vi "initializeArrayElement.vi"(8 "error in (no error)":errorcluster, 9 "arraySize":u16, 10 "arrayRef":refnum<vi>, 11 "Primitive in":refnum<class "Primitive.lvclass">) -> (0 "error out":errorcluster, 3 "Primitive out":refnum<class "Primitive.lvclass">)   [LabVIEW 2012, in "Primitive.lvclass"]
uses:
  Primitive.lvclass
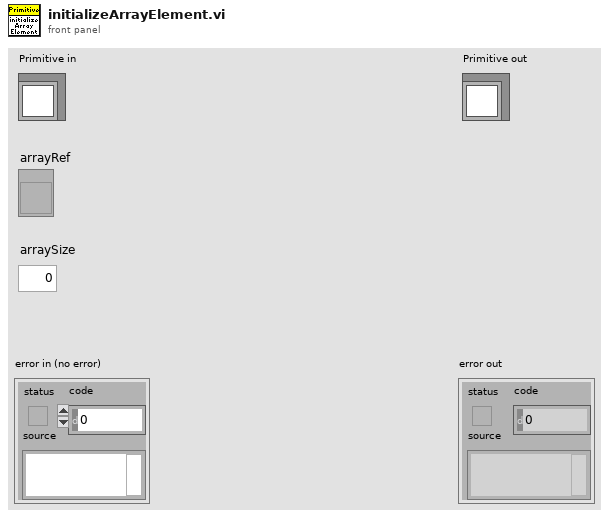
[diagram p1: front panel]
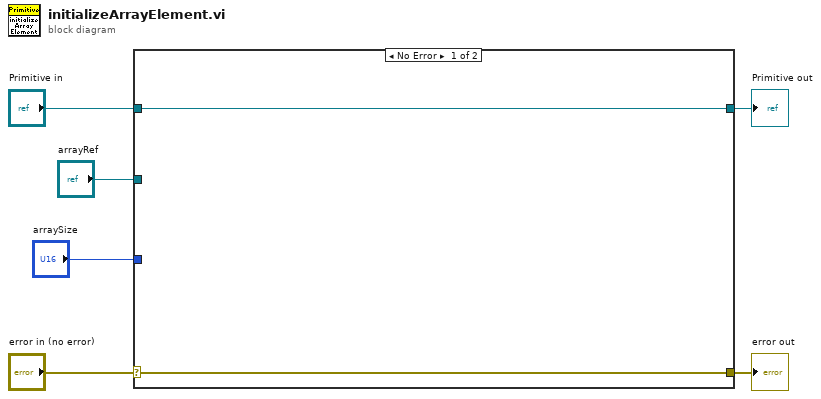
[diagram p0: block diagram]
diagram:
  n1 = case shown="No Error" "error in (no error)" {
    selector: "error in (no error)" -> [w7 w10]
    tunnel: [w7 w10] -> w5
    tunnel: [w8 w9] -> w3
    tunnel: "Primitive in" -> [w8 w9]
    tunnel: "arrayRef" -> [_ _]
    tunnel: "arraySize" -> [_ _]
    frame No Error {
    }
    frame Error {
    }
  }
  "error out" <- w5
  "Primitive out" <- w3
